vi "LoadPuzzleClass.vi"(8 "Error In":errorcluster) -> (0 "Error Out":errorcluster, 2 "PuzzleBase":refnum<class "PuzzleBase.lvclass">)   [LabVIEW 2023, in "AdventCode.lvclass"]
uses:
  AdventCode.lvclass
  PuzzleBase_class/PuzzleBase.lvclass
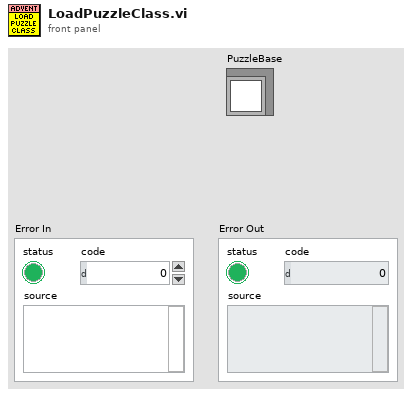
[diagram p1: front panel]
types:
  T1 = typedef "AdventCode.lvclass/ObjectAttributes.ctl" = cluster{"Year":i32, "Day":i32, "PuzzleData":string}
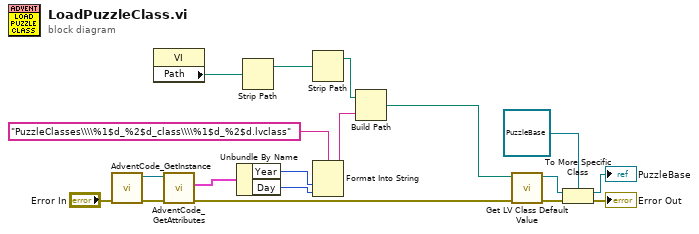
[diagram p0: block diagram]
diagram:
  n1 = call "AdventCode_GetInstance.vi"("error in"="Error In") -> ("error out"=w13:errorcluster, "reference out"=w14:refnum<class "AdventCode.lvclass">)  [unwired: 6 in, 3 out]
  n2 = property class="VI"() -> ("Path"=w12:path)  [unwired: 2 in, 2 out]
  n3 = call "AdventCode_GetAttributes.vi"("error in (no error)"=w13, "reference in"=w14) -> ("error out"=w6:errorcluster, "Data"=w15:T1)  [unwired: 6 in, 2 out]
  n4 = Unbundle By Name(w15) -> ("Year"=w4:i32, "Day"=w3:i32)
  n5 = Strip Path(path=w12) -> (stripped path=w11:path)  [unwired: 1 out]
  n6 = Strip Path(path=w11) -> (stripped path=w10:path)  [unwired: 1 out]
  n7 = Format Into String(format string="PuzzleClasses\\\\%1$d_%2$d_class\\\\%1$d_%2$d.lvclass", w4, w3) -> (resulting string=w2:string)  [unwired: 2 in, 1 out]
  n8 = Build Path(base path=w10, name or relative path=w2) -> (appended path=w1:path)
  n9 = call <vilib>:"Get LV Class Default Value.vi"("error in (no error)"=w6, "class path"=w1) -> ("error out"=w7:errorcluster, "object"=w9:refnum<class>)  [unwired: 8 in]
  n10 = To More Specific Class(target class=refnum<class "PuzzleBase.lvclass"> refnum ("PuzzleBase"), reference=w9, error in=w7) -> (specific class reference=→"PuzzleBase":refnum<class "PuzzleBase.lvclass">, error out=→"Error Out":errorcluster)
